vi "ReCalc_V0.16.vi"(3 "Berechnen":bool, 4 "Datenspeicher":T2={"Fahrzeugdaten"="", "date/time string"="", "Rolle [Inkr/U]"=0, "Rollenumfang [m]"=0.0, "Rollenträgheit [kgm²]"=0.0, "Zündung [Imp/U]"=0, "Getriebe [1:]"=0.0, "Reifenumfang [m] "=0.0, "element"=0.0, "Gl. Mittelwert"=0, "Differenzenquotient"=0, "Polynom"=0, "element"=0.0, "element"=0.0, "Lufttemperatur [°C]"=0.0, "Luftfeuchtigkeit [%]"=0.0, "Luftdruck [mbar]"=0.0, [], [], "Best Polynomial Fit"=[], [], "Übersetzung ermitteln aus"=0, "[s]"=0.0, "nmin [1/min]"=0.0, "nmax [1/min]"=0.0, "n vom Gas [1/min]"=0.0, [], [], "Boolesch"=FALSE, "Serielle Schnittstelle"="COM4"}) -> ()   [LabVIEW 2014]
uses:
  <vilib>/Utility/miscctls.llb/LVPointTypeDef.ctl
  <vilib>/Utility/xml.llb/Read From XML File(string).vi
  <vilib>/Analysis/3filter.llb/IIR Filter (DBL).vi
  <vilib>/Analysis/NI_AALBase.lvlib
  <vilib>/Analysis/NI_AALPro.lvlib
panel:
  out "Fahrzeugdaten":string
  out "Überlagerung":bool
  in  "Überlagern":bool
  out "Übersetzung ermitteln aus":T1(ring)
  in  "Speichern":bool
  out "Reifenumfang [m]":dbl=1.222
  out "Getriebe [1:]":dbl=5.343
  out "Zündung [Imp/U]":u8=1
  out "Rollengeber [Inkr/U]":u16=200
  out "Luftdruck [mbar]":dbl=1013.0
  out "Luftfeuchtigkeit [%]":dbl=50.0
  out "Lufttemperatur [°C]":dbl=20.0
  in  "Stopp":bool
  in  "Rollenträgheit [kgm²]":dbl=0.402
  in  "Polynom":u8=15
  in  "Gl. Mittelwert":u8=35
  in  "Differenzenquotient":u8=12
  in  "n vom Gas [1/min]":dbl=5000.0
  out "Rollenumfang [m]":dbl=0.613 format="%.3f"
  out "Datum, Zeit":string
  out "Untersetzung aus:":dbl=2.68 format="%.2f"
  in  "Drucken":bool
  out "Pmax":string
  out "Ergebnis":string
  out "XY-Graph":cluster{dbl[], dbl[]}[](graph)
  in  "Öffnen":bool
  out "korr":dbl
  out "[s]":dbl=5.0
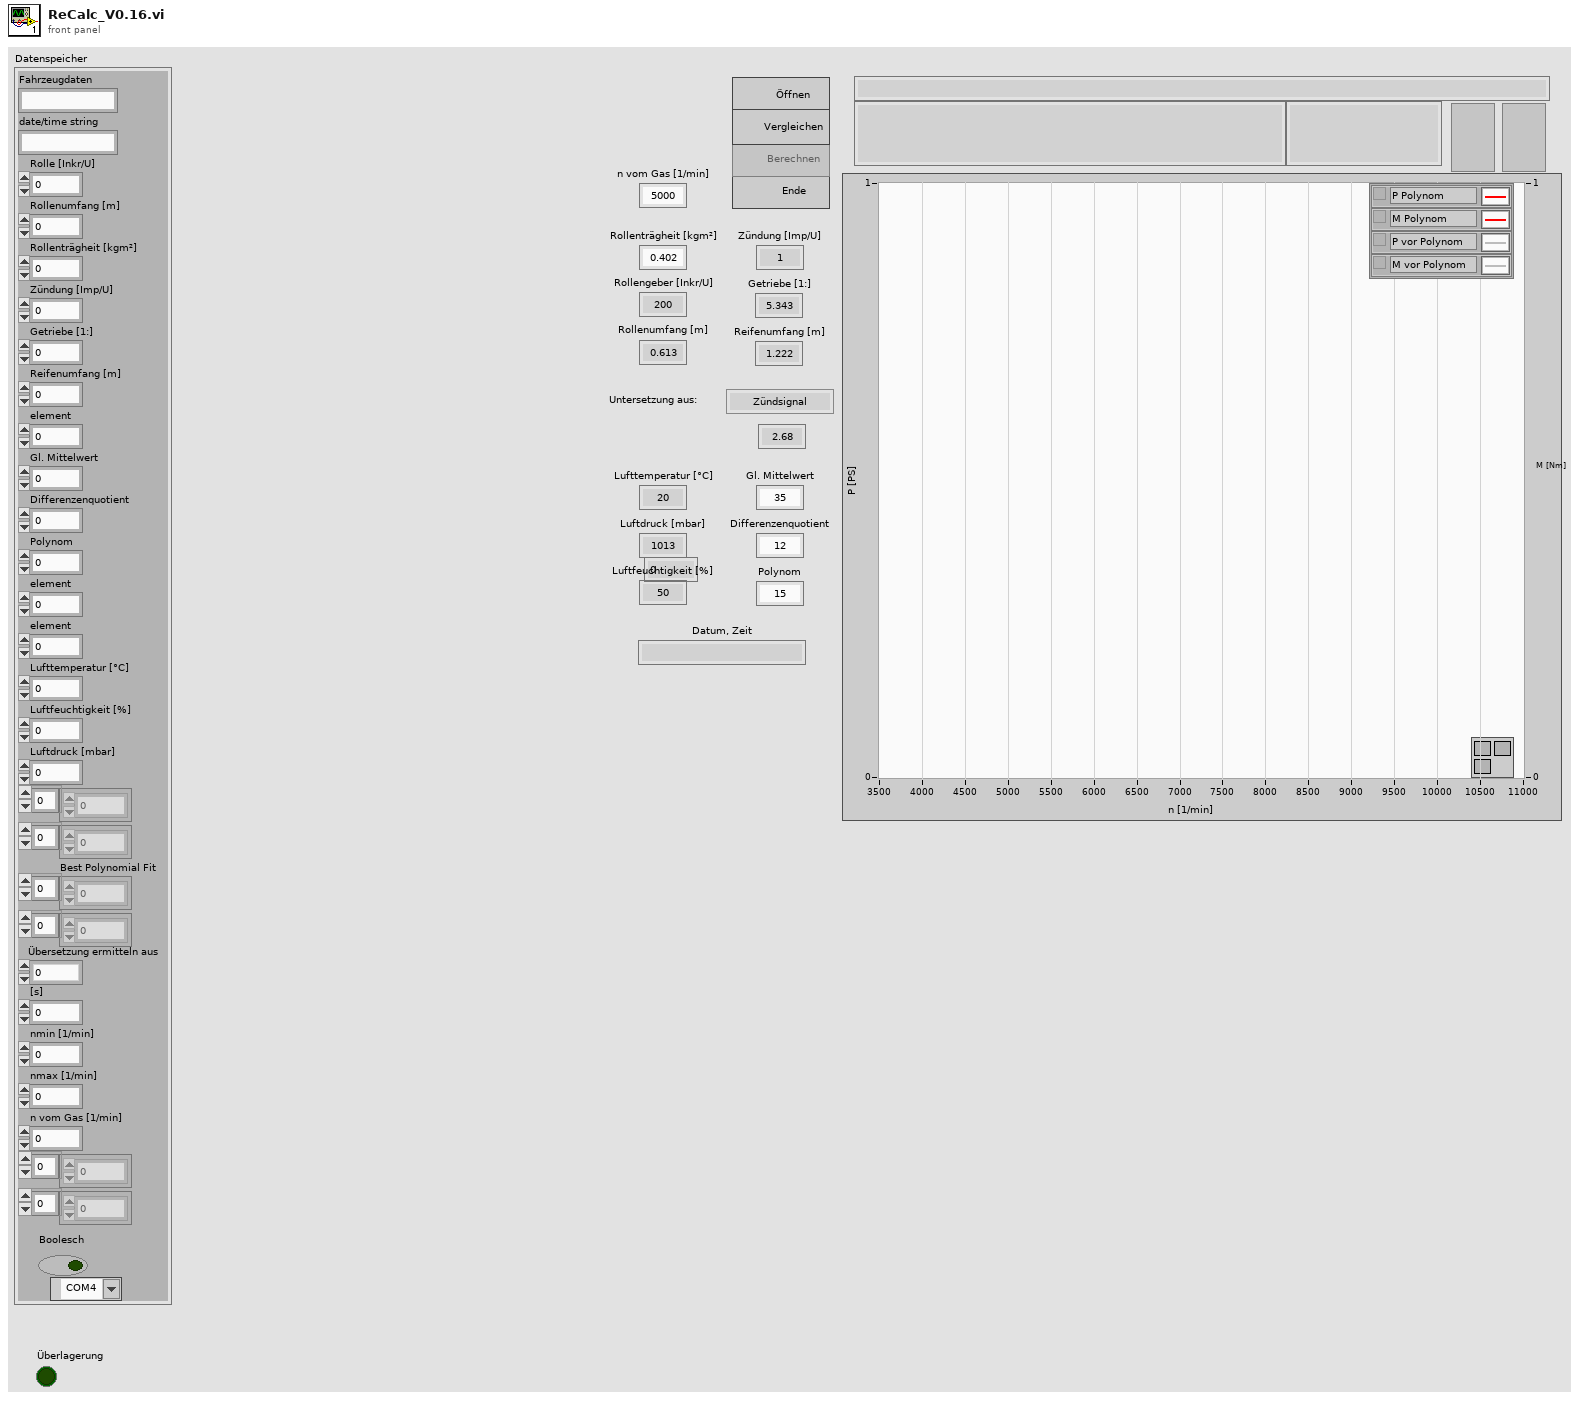
[diagram p1: front panel]
types:
  T1 = enum8{"Zündsignal", "Getriebe & Reifen", "nKuWe / nRolle :"}
  T2 = cluster{"Fahrzeugdaten":string, "date/time string":string, "Rolle [Inkr/U]":u16, "Rollenumfang [m]":dbl, "Rollenträgheit [kgm²]":dbl, "Zündung [Imp/U]":u8, "Getriebe [1:]":dbl, "Reifenumfang [m] ":dbl, "element":dbl, "Gl. Mittelwert":u8, "Differenzenquotient":u8, "Polynom":u8, "element":dbl, "element":dbl, "Lufttemperatur [°C]":dbl, "Luftfeuchtigkeit [%]":dbl, "Luftdruck [mbar]":dbl, dbl[], dbl[], "Best Polynomial Fit":dbl[], dbl[], "Übersetzung ermitteln aus":u8, "[s]":dbl, "nmin [1/min]":dbl, "nmax [1/min]":dbl, "n vom Gas [1/min]":dbl, dbl[], i32[], "Boolesch":bool, "Serielle Schnittstelle":refnum<visa-resource-name>}
  T3 = typedef "LVPointTypeDef.ctl" = cluster{"Horizontal":i16, "Vertical":i16}
  T4 = enum16{"Kleinste Quadrate", "Kleinestes absolutes Reiduum", "Biquadrat"}
  T5 = enum8{"Enabled", "Disabled", "Disabled and Grayed Out"}
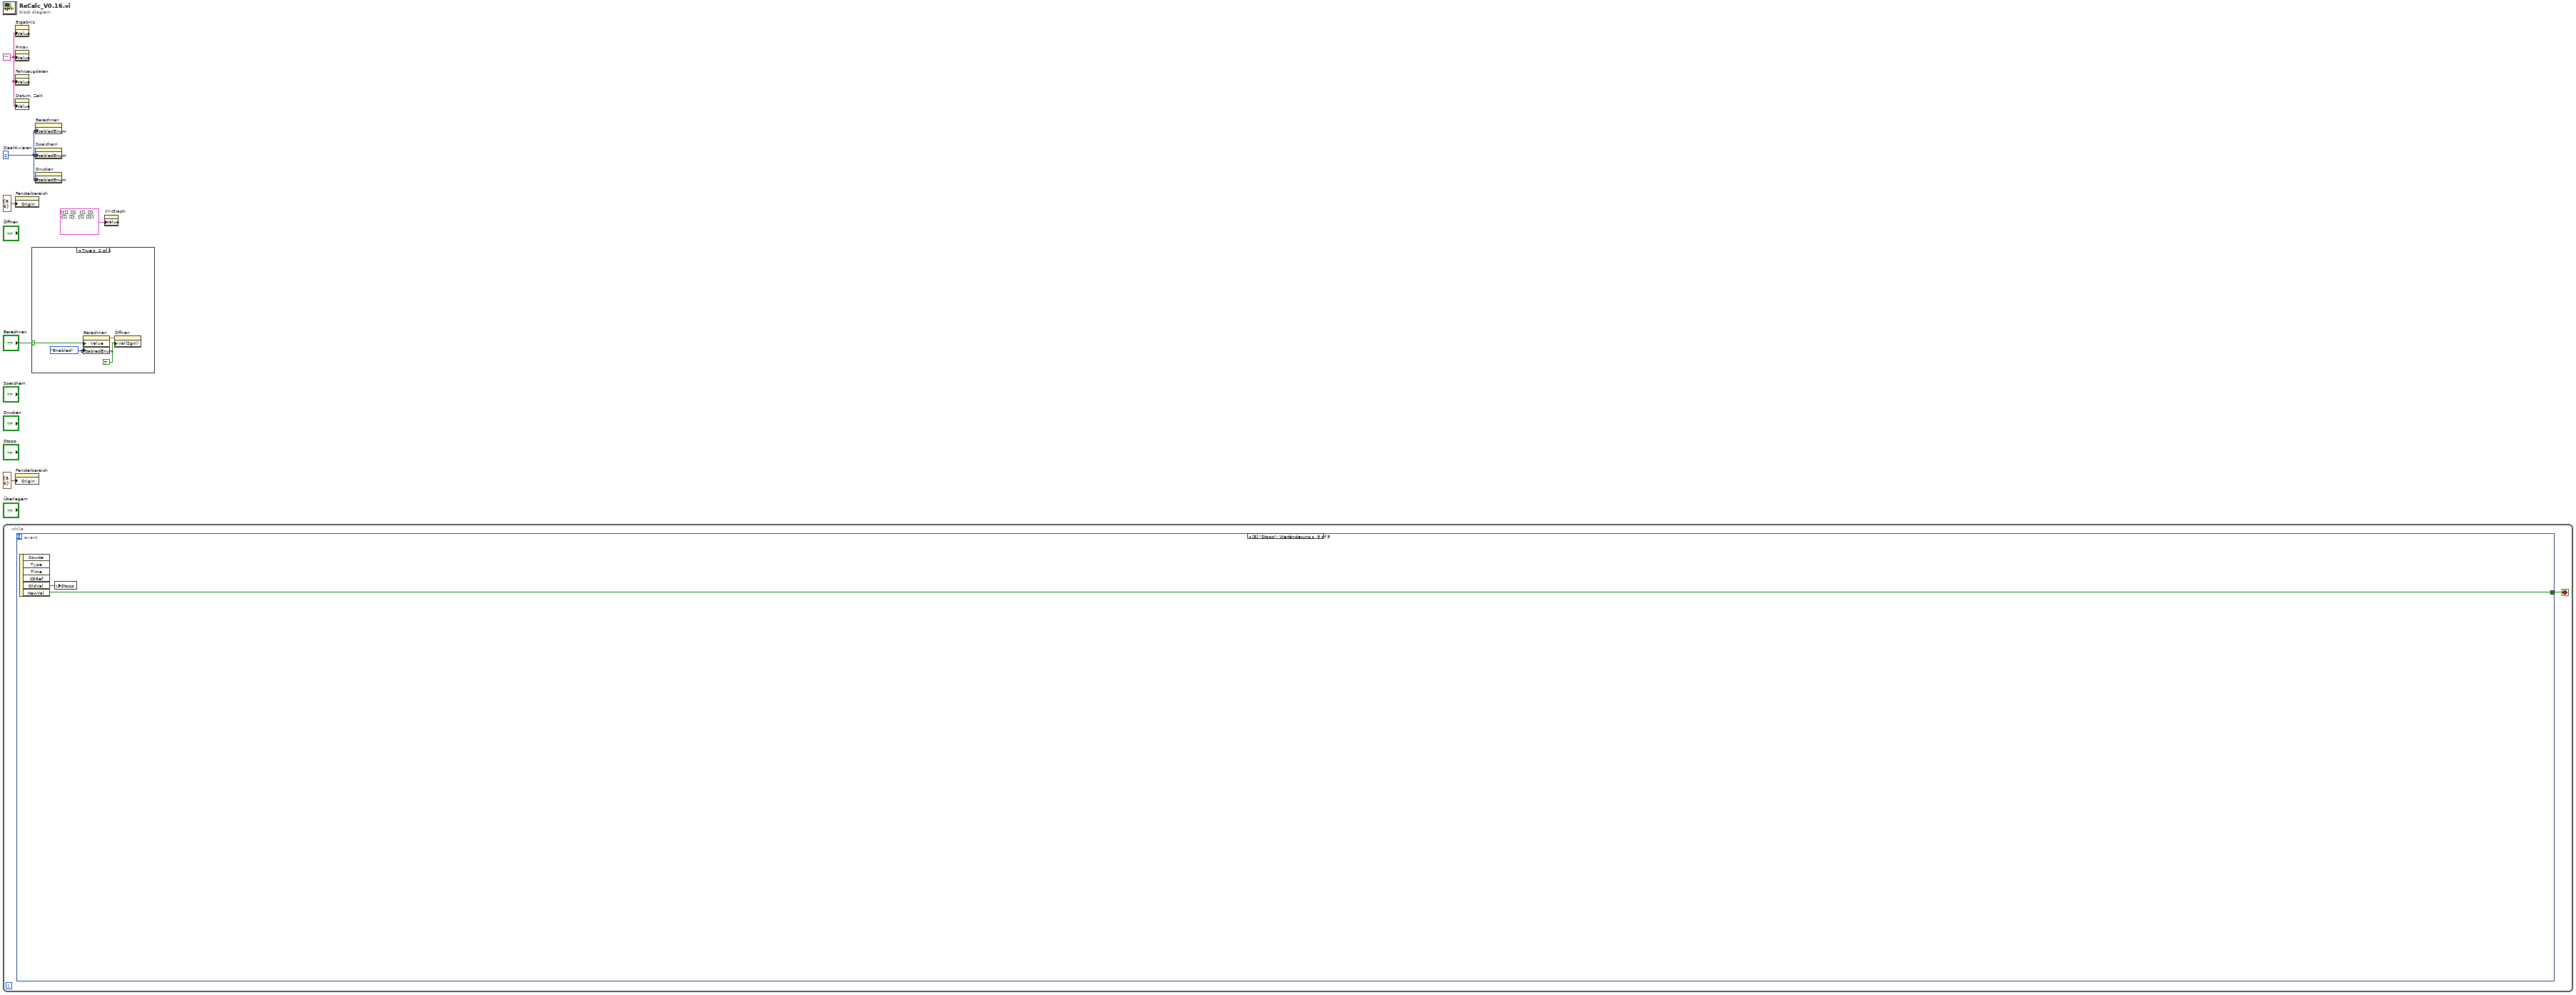
[diagram p0: block diagram]
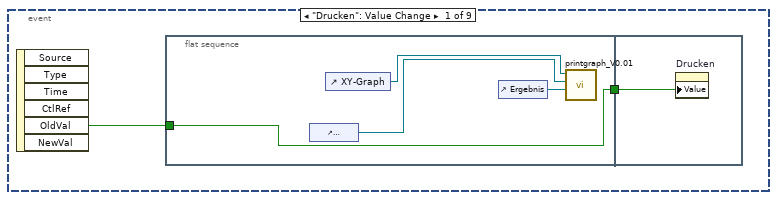
[diagram p3: hidden frame]
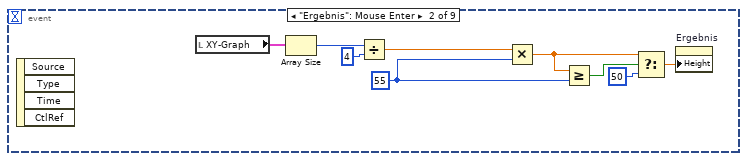
[diagram p4: hidden frame]
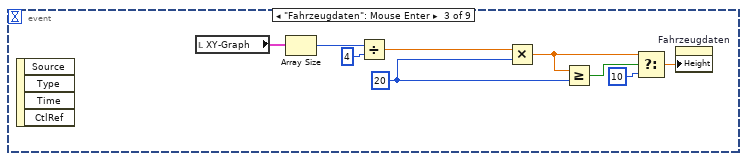
[diagram p5: hidden frame]
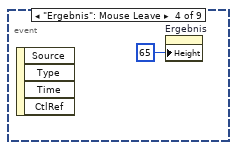
[diagram p6: hidden frame]
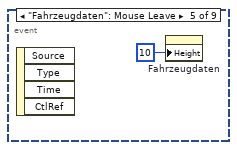
[diagram p7: hidden frame]
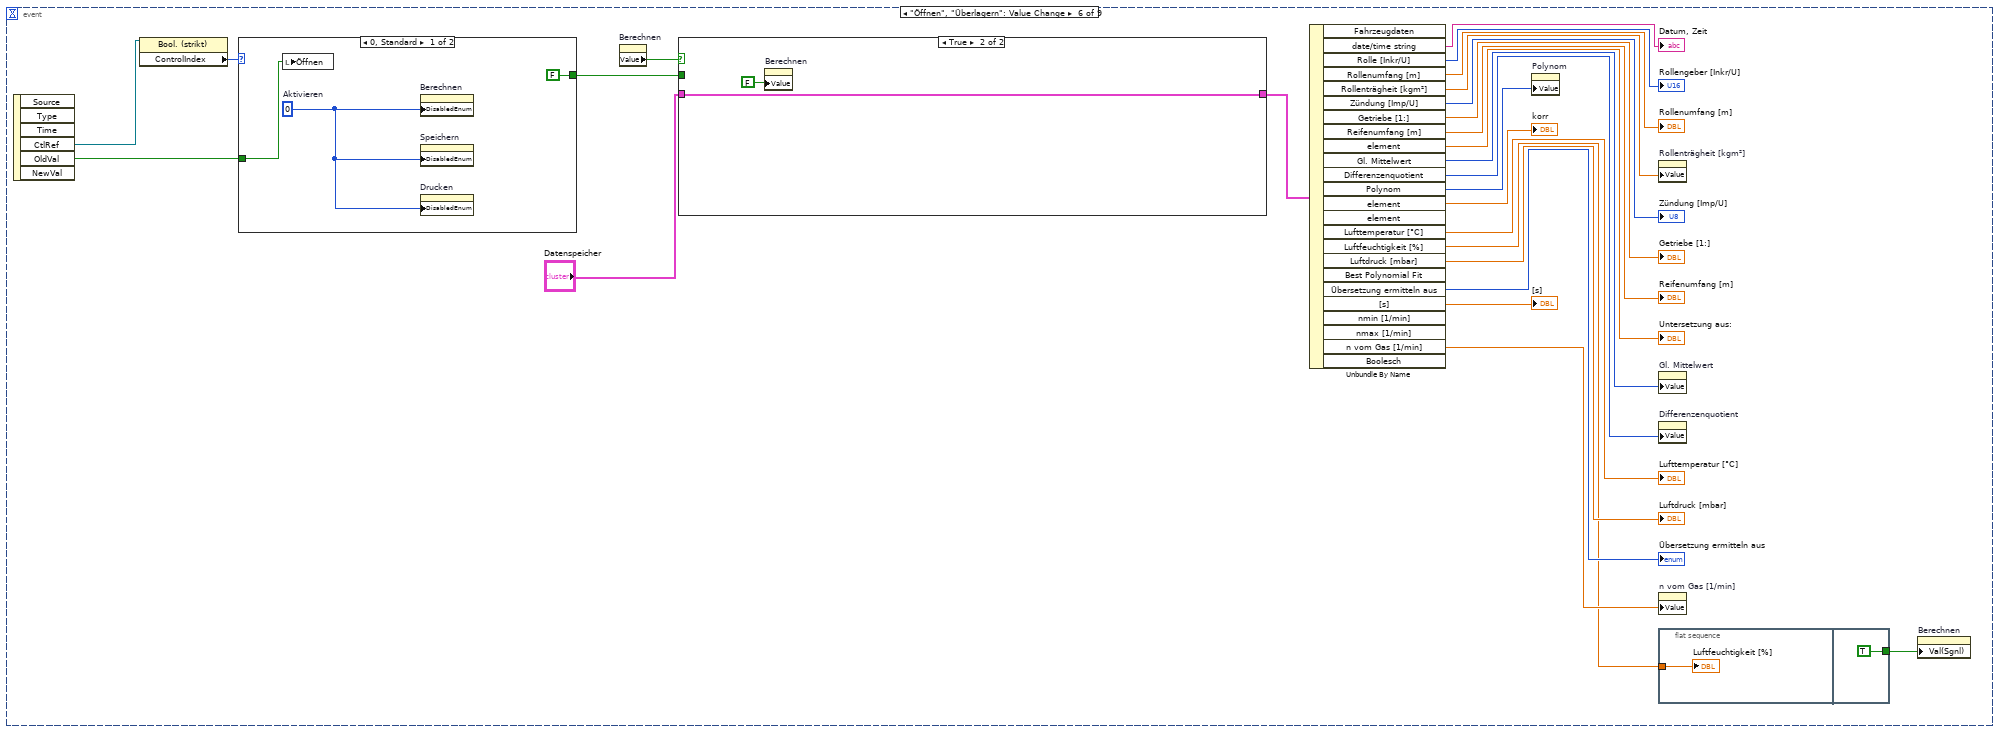
[diagram p8: hidden frame]
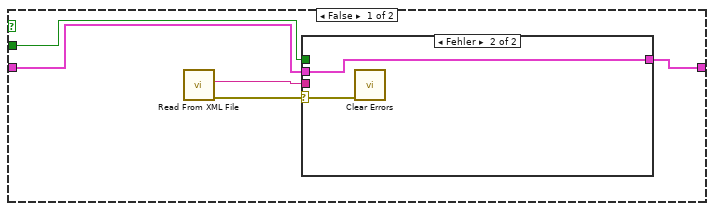
[diagram p9: hidden frame]
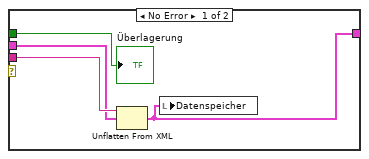
[diagram p10: hidden frame]
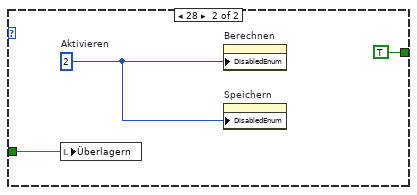
[diagram p11: hidden frame]
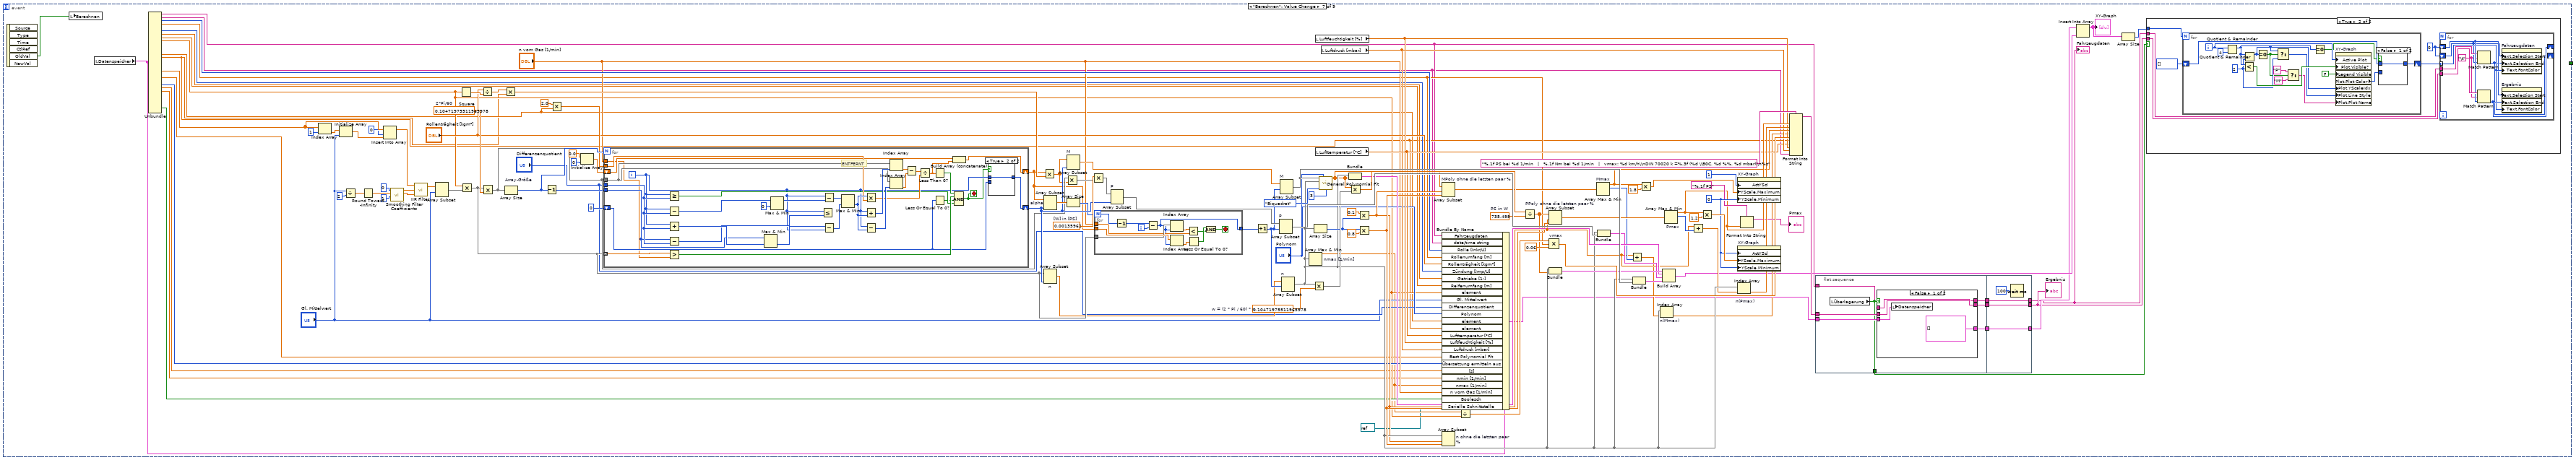
[diagram p12: hidden frame]
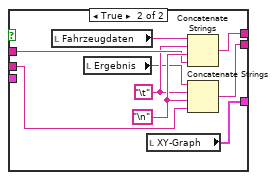
[diagram p13: hidden frame]
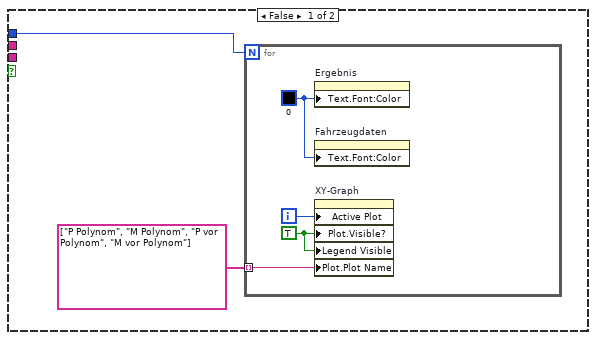
[diagram p14: hidden frame]
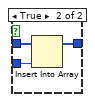
[diagram p15: hidden frame]
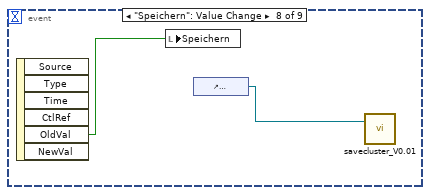
[diagram p17: hidden frame]
diagram:
  w4 = 2  # Deaktivieren
  w6 = ""
  n1 = while {
    stop <- w7 stop-if-true
    n2 = event shown="[8] \"Stopp\": Wertänderung" {
      selector: _ -> [_ _ _ _ _ _ _ _ _]
      dyn-events: _ -> [_ _ _ _ _ _ _ _ _]
      timeout: _ -> [_ _ _ _ _ _ _ _ _]
      tunnel: [_ _ _ _ _ _ _ _ w318] -> w7
      event "Drucken": Value Change {
        n3 = event-data() -> ("OldVal"=w9:bool)  [unwired: 1 in, 5 out]
        n4 = flat-sequence {
          tunnel: w9 -> [w13]
          tunnel: [w13] -> w8
          tunnel: w8 -> [w14]
          frame #0 {
            n5 = control-ref of="Fahrzeugdaten"() -> (w11:refnum<vi>)
            n6 = control-ref of="XY-Graph"() -> (w12:refnum<vi>)
            n7 = control-ref of="Ergebnis"() -> (w10:refnum<vi>)
            n8 = call "printgraph_V0.01.vi"("reference 2"=w10, "Fahrzeugdaten"=w11, "XYGraph (Eingang)"=w12) -> ()  [unwired: 9 in]
          }
          frame #1 {
            n9 = property on="Drucken" class="Bool. (strikt)"("Value"=w14) -> ()  [unwired: 2 in, 2 out]
          }
        }
      }
      event "Ergebnis": Mouse Enter {
        w17 = u32 55 ("Größe:Höhe")
        n10 = event-data() -> ()  [unwired: 1 in, 4 out]
        n11 = local read "XY-Graph"() -> (w23:cluster{dbl[], dbl[]}[])
        n12 = Array Size(array=w23) -> (size(s)=w22:i32)
        n13 = Divide(x=w22, y=4) -> (x/y=w20:dbl)
        n14 = Multiply(x=w20, y=w17) -> (x*y=w18:dbl)
        n15 = Greater Or Equal?(x=w18, y=w17) -> (x >= y?=w19:bool)
        n16 = Select(t=w18, s=w19, f=u32 50 ("Größe:Höhe")) -> (s? t:f=w16:dbl)
        n17 = property on="Ergebnis" class="Str"("Height"=w16) -> ()  [unwired: 2 in, 2 out]
      }
      event "Fahrzeugdaten": Mouse Enter {
        w26 = u32 20 ("Größe:Höhe")
        n18 = event-data() -> ()  [unwired: 1 in, 4 out]
        n19 = local read "XY-Graph"() -> (w32:cluster{dbl[], dbl[]}[])
        n20 = Array Size(array=w32) -> (size(s)=w31:i32)
        n21 = Divide(x=w31, y=4) -> (x/y=w29:dbl)
        n22 = Multiply(x=w29, y=w26) -> (x*y=w27:dbl)
        n23 = Greater Or Equal?(x=w27, y=w26) -> (x >= y?=w28:bool)
        n24 = Select(t=w27, s=w28, f=u32 10 ("Größe:Höhe")) -> (s? t:f=w25:dbl)
        n25 = property on="Fahrzeugdaten" class="Str"("Height"=w25) -> ()  [unwired: 2 in, 2 out]
      }
      event "Ergebnis": Mouse Leave {
        n26 = event-data() -> ()  [unwired: 1 in, 4 out]
        n27 = property on="Ergebnis" class="Str"("Height"=u32 65 ("Größe:Höhe")) -> ()  [unwired: 2 in, 2 out]
      }
      event "Fahrzeugdaten": Mouse Leave {
        n28 = event-data() -> ()  [unwired: 1 in, 4 out]
        n29 = property on="Fahrzeugdaten" class="Str"("Height"=u32 10 ("Größe:Höhe")) -> ()  [unwired: 2 in, 2 out]
      }
      event "Öffnen", "Überlagern": Value Change {
        n30 = event-data() -> ("CtlRef"=w59:refnum<vi>, "OldVal"=w57:bool)  [unwired: 1 in, 4 out]
        n31 = property class="Bool. (strikt)"(reference=w59) -> ("ControlIndex"=w58:i32)  [unwired: 1 in, 2 out]
        n32 = case shown="0, Standard" w58 {
          tunnel: w57 -> [w78 w81]
          tunnel: [FALSE ("Überlagerung") TRUE ("Überlagerung")] -> w56
          frame 0, Default {
            w76 = 0  # Aktivieren
            n33 = local write "Öffnen"(w78) -> ()
            n34 = property on="Berechnen" class="Bool. (strikt)"("DisabledEnum"=w76) -> ()  [unwired: 2 in, 2 out]
            n35 = property on="Speichern" class="Bool. (strikt)"("DisabledEnum"=w76) -> ()  [unwired: 2 in, 2 out]
            n36 = property on="Drucken" class="Bool. (strikt)"("DisabledEnum"=w76) -> ()  [unwired: 2 in, 2 out]
          }
          frame 28 {
            w79 = 2  # Aktivieren
            n37 = local write "Überlagern"(w81) -> ()
            n38 = property on="Berechnen" class="Bool. (strikt)"("DisabledEnum"=w79) -> ()  [unwired: 2 in, 2 out]
            n39 = property on="Speichern" class="Bool. (strikt)"("DisabledEnum"=w79) -> ()  [unwired: 2 in, 2 out]
          }
        }
        n40 = property on="Berechnen" class="Bool. (strikt)"() -> ("Value"=w35:bool)  [unwired: 2 in, 2 out]
        n41 = case shown="True" w35 {
          tunnel: "Datenspeicher" -> [w64 w72]
          tunnel: w56 -> [w62 _]
          tunnel: [w61 w72] -> w36
          frame False {
            n42 = call-poly <vilib>:"Read From XML File.vi"() -> ("error out"=w63:errorcluster, "XML Elements"=w65:string)  [unwired: 9 in, 1 out]
            n43 = case shown="Fehler" w63 {
              selector: w63 -> [_ w71]
              tunnel: w65 -> [w69 _]
              tunnel: w64 -> [w67 w70]
              tunnel: w62 -> [w68 _]
              tunnel: [w66 w70] -> w61
              frame No Error {
                n44 = Unflatten From XML(xml string=w69, type=w67) -> (value=w66:T2)  [unwired: 1 in, 1 out]
                n45 = local write "Datenspeicher"(w66) -> ()
                "Überlagerung" <- w68
              }
              frame Error {
                n46 = call <vilib>:"Clear Errors.vi"("error in (no error)"=w71) -> ()  [unwired: 5 in, 2 out]
              }
            }
          }
          frame True {
            n47 = property on="Berechnen" class="Bool. (strikt)"("Value"=FALSE) -> ()  [unwired: 2 in, 2 out]
          }
        }
        n48 = Unbundle By Name(w36) -> ("date/time string"=→"Datum, Zeit":string, "Rolle [Inkr/U]"=→"Rollengeber [Inkr/U]":u16, "Rollenumfang [m]"=→"Rollenumfang [m]":dbl, "Rollenträgheit [kgm²]"=w41:dbl, "Zündung [Imp/U]"=→"Zündung [Imp/U]":u8, "Getriebe [1:]"=→"Getriebe [1:]":dbl, "Reifenumfang [m]"=→"Reifenumfang [m]":dbl, "element"=→"Untersetzung aus:":dbl, "Gl. Mittelwert"=w46:u8, "Differenzenquotient"=w47:u8, "Polynom"=w48:u8, "element"=→"korr":dbl, "Lufttemperatur [°C]"=→"Lufttemperatur [°C]":dbl, "Luftfeuchtigkeit [%]"=w51:dbl, "Luftdruck [mbar]"=→"Luftdruck [mbar]":dbl, "Übersetzung ermitteln aus"=→"Übersetzung ermitteln aus":u8, "[s]"=→"[s]":dbl, "n vom Gas [1/min]"=w55:dbl)  [unwired: 6 out]
        n49 = property on="Polynom" class="DigWert (strikt)"("Value"=w48) -> ()  [unwired: 2 in, 2 out]
        n50 = property on="Rollenträgheit [kgm²]" class="DigWert (strikt)"("Value"=w41) -> ()  [unwired: 2 in, 2 out]
        n51 = property on="Gl. Mittelwert" class="DigWert (strikt)"("Value"=w46) -> ()  [unwired: 2 in, 2 out]
        n52 = property on="Differenzenquotient" class="DigWert (strikt)"("Value"=w47) -> ()  [unwired: 2 in, 2 out]
        n53 = property on="n vom Gas [1/min]" class="DigWert (strikt)"("Value"=w55) -> ()  [unwired: 2 in, 2 out]
        n54 = flat-sequence {
          tunnel: w51 -> [w74]
          tunnel: [TRUE] -> w37
          frame #0 {
            "Luftfeuchtigkeit [%]" <- w74
          }
          frame #1 {
          }
        }
        n55 = property on="Berechnen" class="Bool. (strikt)"("Val(Sgnl)"=w37) -> ()  [unwired: 2 in, 2 out]
      }
      event "Berechnen": Value Change {
        w165 = 0
        w173 = 735.498  # PS in W
        w178 = 0.10471975511965978  # w = (2 * Pi / 60) * n
        w189 = 0.00135962  # [W] in [PS]
        w198 = 0.10471975511965978  # 2*Pi/60
        n56 = event-data() -> ("OldVal"=w95:bool)  [unwired: 1 in, 5 out]
        n57 = local write "Berechnen"(w95) -> ()
        n58 = local read "Datenspeicher"() -> (w121:T2)
        n59 = Unbundle(w121) -> ("Fahrzeugdaten"=w87:string, "date/time string"=w86:string, "Rolle [Inkr/U]"=w117:u16, "Rollenumfang [m]"=w108:dbl, "Zündung [Imp/U]"=w107:u8, "Getriebe [1:]"=w106:dbl, "Reifenumfang [m]"=w105:dbl, "element"=w104:dbl, "element"=w103:dbl, "element"=w102:dbl, w204:dbl[], "Best Polynomial Fit"=w101:dbl[], "Übersetzung ermitteln aus"=w109:u8, "[s]"=w98:dbl, "nmin [1/min]"=w99:dbl, "Boolesch"=w112:bool)  [unwired: 14 out]
        n60 = Index Array(array=w204, index=1) -> (element=w127:dbl)
        n61 = Initialize Array(w127, "Gl. Mittelwert") -> (w128:dbl[])
        n62 = Divide(x="Gl. Mittelwert", y=2) -> (x/y=w201:dbl)
        n63 = Round Toward -Infinity(1:w201) -> (0:w200:dbl)
        n64 = Insert Into Array ("In Array einfügen")(array=w204, index=0, new element=w128) -> (w125:dbl[])
        n65 = call <vilib>:"Smoothing Filter Coefficients.vi"("shape"=1, "half-width"=w200, "type"=0) -> ("forward coefficients"=w129:dbl[], "reverse coefficients"=w130:dbl[])  [unwired: 6 in, 1 out]
        n66 = call-poly <vilib>:"IIR Filter.vi"("Forward Coefficients"=w129, "Reverse Coefficients"=w130, "X"=w125) -> ("Filtered X"=w124:dbl[])  [unwired: 1 in, 1 out]
        n67 = Array Subset(array=w124, index="Gl. Mittelwert") -> (w123:dbl[])  [unwired: 1 in]
        n68 = Square(x=w104) -> (x^2=w190:dbl)
        n69 = Multiply(x=w104, y=w123) -> (x*y=w132:dbl[])
        n70 = Divide(x="Rollenträgheit [kgm²]", y=w190) -> (x/y=w187:dbl)
        n71 = Multiply(x=w132, y=w198) -> (x*y=w155:dbl[])
        n72 = Multiply(x=w187, y=w102) -> (x*y=w186:dbl)
        n73 = Array Size "Array-Größe"(array=w155) -> (size(s)=w196:i32)
        n74 = Decrement(x=w196) -> (x-1=w197:i32)
        n75 = Multiply(x=2.0, y=w103) -> (x*y=w195:dbl)
        n76 = Initialize Array(0.0 ("y"), 0) -> (w191:dbl[])
        n77 = for {
          N: w196 -> [_]
          tunnel: "Differenzenquotient" -> [w291]
          tunnel: w155 -> [w298]
          tunnel: w197 -> [w290]
          tunnel: w195 -> [w299]
          shift-right: [w295] -> w154
          shift-left: w191 -> [w296]
          tunnel: w132 -> [w293] mode=indexing
          tunnel: "n vom Gas [1/min]" -> [w282]
          shift-right: [w281] -> w182
          shift-left: 0 -> [w284]
          i -> [w285]
          stop <- w283 stop-if-true
          # "ENTFERNT"
          n78 = Greater Or Equal?(x=w285, y=w291) -> (x >= y?=w288:bool)
          n79 = Subtract(x=w285, y=w291) -> (x-y=w312:i32)
          n80 = Add(x=w285, y=w291) -> (x+y=w306:i32)
          n81 = Subtract(x=w290, y=w291) -> (x-y=w292:i32)
          n82 = Greater?(x=w293, y=w282) -> (0:w294:bool)
          n83 = Max & Min(x=w290, y=w306) -> (min(x,y)=w307:i32)  [unwired: 1 out]
          n84 = Max & Min(x=w312, y=0) -> (max(x,y)=w310:i32)  [unwired: 1 out]
          n85 = Less Or Equal?(x=w285, y=w292) -> ()  [unwired: 1 out]
          n86 = Subtract(x=w285, y=w310) -> (x-y=w309:i32)
          n87 = Subtract(x=w307, y=w285) -> (x-y=w308:i32)
          n88 = Max & Min(x=w309, y=w308) -> (min(x,y)=w300:i32)  [unwired: 1 out]
          n89 = Multiply(x=w300, y=w299) -> (x*y=w297:dbl)
          n90 = Add(x=w285, y=w300) -> (x+y=w305:i32)
          n91 = Subtract(x=w285, y=w300) -> (x-y=w304:i32)
          n92 = Index Array(array=w298, index=w305) -> (element=w302:dbl)
          n93 = Index Array(array=w298, index=w304) -> (element=w303:dbl)
          n94 = Subtract(x=w302, y=w303) -> (x-y=w301:dbl)
          n95 = Divide(x=w301, y=w297) -> (x/y=w289:dbl)
          n96 = Less Than 0?(x=w289) -> (x < 0?=w287:bool)
          n97 = Less Or Equal To 0?(x=w284) -> (x <= 0?=w286:bool)
          n98 = Build Array (concatenate)(w296, w289) -> (w295:dbl[])
          n99 = Compound Arithmetic op=AND(w287, w294, w286, w288) -> (w283:bool)
          n100 = case shown="True" w283 {
            tunnel: w285 -> [_ w314]
            tunnel: [w313 w314] -> w281
            tunnel: w284 -> [w313 _]
            frame False {
            }
            frame True {
            }
          }
        }
        n101 = Multiply(x=w154, y=w186) -> (x*y=w152:dbl[])
        n102 = Array Subset "alpha"(array=w154, length=w182) -> (w184:dbl[])  [unwired: 1 in]
        n103 = Array Subset "n"(array=w132, length=w182) -> (w131:dbl[])  [unwired: 1 in]
        n104 = Multiply(x=w155, y=w152) -> (x*y=w188:dbl[])
        n105 = Array Subset "M"(array=w152, length=w182) -> (w153:dbl[])  [unwired: 1 in]
        n106 = Array Size(array=w184) -> (size(s)=w181:i32)
        n107 = Multiply(x=w189, y=w188) -> (x*y=w183:dbl[])
        n108 = for {
          N: w181 -> [w280]
          tunnel: w154 -> [w277]
          tunnel: w132 -> [w274]
          tunnel: "n vom Gas [1/min]" -> [w271]
          tunnel: [w269] -> w180
          i -> [w275]
          stop <- w270 stop-if-true
          n109 = Decrement(x=w280) -> (x-1=w279:i32)
          n110 = Subtract(x=w279, y=w275) -> (x-y=w269:i32)
          n111 = Index Array(array=w274, index=w269) -> (element=w273:dbl)
          n112 = Index Array(array=w277, index=w269) -> (element=w278:dbl)
          n113 = Less?(x=w273, y=w271) -> (x < y?=w272:bool)
          n114 = Less Or Equal To 0?(x=w278) -> (x <= 0?=w276:bool)
          n115 = And(x=w276, y=w272) -> (x .and. y?=w270:bool)
        }
        n116 = Array Subset "P"(array=w183, length=w182) -> (w172:dbl[])  [unwired: 1 in]
        n117 = Increment(x=w180) -> (x+1=w171:i32)
        n118 = Array Subset "P"(array=w172, index=w171) -> (w179:dbl[])  [unwired: 1 in]
        n119 = Array Subset "M"(array=w153, index=w171) -> (w177:dbl[])  [unwired: 1 in]
        n120 = Array Subset "n"(array=w131, index=w171) -> (w140:dbl[])  [unwired: 1 in]
        n121 = Array Max & Min "nmax [1/min]"(array=w140) -> (max value=w100:dbl)  [unwired: 3 out]
        n122 = Multiply(x=w140, y=w178) -> (x*y=w164:dbl[])
        n123 = Array Size(array=w140) -> (size(s)=w142:i32)
        n124 = local read "Luftfeuchtigkeit [%]"() -> (w119:dbl)
        n125 = local read "Lufttemperatur [°C]"() -> (w118:dbl)
        n126 = call <vilib>:"General Polynomial Fit.vi"("Y"=w177, "polynomial order"="Polynom", "X"=w140, "method"=T4."Biquadrat" ("Methode"), "algorithm"=3) -> ("Best Polynomial Fit"=w139:dbl[])  [unwired: 7 in, 3 out]
        n127 = local read "Luftdruck [mbar]"() -> (w120:dbl)
        n128 = Bundle(w140, "Best Polynomial Fit"=w139) -> (w150:cluster{dbl[], "Best Polynomial Fit":dbl[]})  [unwired: 1 in]
        n129 = Multiply(x=w139, y=w164) -> (x*y=w174:dbl[])
        n130 = Multiply(x=0.1, y=w142) -> (x*y=w135:dbl)
        n131 = Multiply(x=w142, y=0.8) -> (x*y=w143:dbl)
        n132 = Array Subset "MPoly ohne die letzten paar %"(array=w139, index=w135, length=w143) -> (w144:dbl[])
        n133 = Bundle By Name(cluster=w121, "Fahrzeugdaten"=w87, "date/time string"=w86, "Rolle [Inkr/U]"=w117, "Rollenumfang [m]"=w108, "Rollenträgheit [kgm²]"="Rollenträgheit [kgm²]", "Zündung [Imp/U]"=w107, "Getriebe [1:]"=w106, "Reifenumfang [m]"=w105, "element"=w104, "Gl. Mittelwert"="Gl. Mittelwert", "Differenzenquotient"="Differenzenquotient", "Polynom"="Polynom", "element"=w103, "element"=w102, "Lufttemperatur [°C]"=w118, "Luftfeuchtigkeit [%]"=w119, "Luftdruck [mbar]"=w120, "Best Polynomial Fit"=w101, "Übersetzung ermitteln aus"=w109, "[s]"=w98, "nmin [1/min]"=w99, "nmax [1/min]"=w100, "n vom Gas [1/min]"="n vom Gas [1/min]", "Boolesch"=w112, "Serielle Schnittstelle"=refnum<visa-resource-name> refnum) -> (w93:T2)
        n134 = Array Subset "n ohne die letzten paar %"(array=w140, index=w135, length=w143) -> ()  [unwired: 1 out]
        n135 = Divide(x=w100, y=w104) -> (x/y=w163:dbl)
        n136 = Divide(x=w174, y=w173) -> (x/y=w138:dbl[])
        n137 = Array Subset "PPoly ohne die letzten paar %"(array=w138, index=w135, length=w143) -> (w145:dbl[])
        n138 = Compound Arithmetic op=MULTIPLY "vmax"(w163, w108, 0.06) -> (w160:dbl)
        n139 = Bundle(w140, w138) -> (w151:cluster{dbl[], dbl[]})  [unwired: 1 in]
        n140 = Array Max & Min "Mmax"(array=w144) -> (max value=w157:dbl, max index (indices)=w136:i32)  [unwired: 2 out]
        n141 = Bundle(w140, w179) -> (w149:cluster{dbl[], dbl[]})  [unwired: 1 in]
        n142 = Add(x=w135, y=w136) -> (x+y=w134:dbl)
        n143 = Bundle(w140, w177) -> (w148:cluster{dbl[], dbl[]})  [unwired: 1 in]
        n144 = Multiply(x=w157, y=1.8) -> (x*y=w166:dbl)
        n145 = Index Array "n(Mmax)"(array=w140, index=w134) -> (element=w110:dbl)
        n146 = Build Array(w151, w150, w149, w148) -> (w91:cluster{dbl[], "Best Polynomial Fit":dbl[]}[])
        n147 = Array Max & Min "Pmax"(array=w145) -> (max value=w158:dbl, max index (indices)=w137:i32)  [unwired: 2 out]
        n148 = Add(x=w135, y=w137) -> (x+y=w133:dbl)
        n149 = Multiply(x=w158, y=1.2) -> (x*y=w167:dbl)
        n150 = property on="XY-Graph" class="XYGraph (strikt)"("ActYScl"=1, "YScale.Maximum"=w166, "YScale.Minimum"=w165) -> ()  [unwired: 2 in, 2 out]
        n151 = property on="XY-Graph" class="XYGraph (strikt)"("ActYScl"=w165, "YScale.Maximum"=w167, "YScale.Minimum"=w165) -> ()  [unwired: 2 in, 2 out]
        n152 = Index Array "n(Pmax)"(array=w140, index=w133) -> (element=w161:dbl)
        n153 = Format Into String(format string="%.1f PS" ("Format-String"), w158) -> (resulting string=→"Pmax":string)  [unwired: 2 in, 1 out]
        n154 = Format Into String(format string="%.1f PS bei %d 1/min   |   %.1f Nm bei %d 1/min   |   vmax: %d km/h\\nDIN 70020 k =%.3f (%d \\B0C, %d %%, %d mbar)\\n%s" ("Format-String"), w158, w161, w157, w110, w160, w102, w118, w119, w120, w86) -> (resulting string=w97:string)  [unwired: 2 in, 1 out]
        n155 = flat-sequence {
          tunnel: w97 -> [w211]
          tunnel: w93 -> [w210]
          tunnel: [w209] -> w92
          tunnel: w87 -> [w205]
          tunnel: [w208] -> w85
          tunnel: [w207] -> w84
          tunnel: [w206] -> w83
          tunnel: [w226] -> w88
          tunnel: [w227] -> w89
          tunnel: [w228] -> w90
          tunnel: w85 -> [w228]
          tunnel: w84 -> [w227]
          tunnel: w83 -> [w226]
          frame #0 {
            n156 = local read "Überlagerung"() -> (w209:bool)
            n157 = case shown="False" w209 {
              tunnel: [cluster{dbl[], dbl[]}[] [] ("XY-Graph") w224] -> w208
              tunnel: w211 -> [w214 w222]
              tunnel: [w214 w223] -> w207
              tunnel: w210 -> [w213 _]
              tunnel: w205 -> [w212 w220]
              tunnel: [w212 w219] -> w206
              frame False {
                n158 = local write "Datenspeicher"(w213) -> ()
              }
              frame True {
                w218 = "\t"
                w221 = "\n"
                n159 = local read "Fahrzeugdaten"() -> (w217:string)
                n160 = local read "Ergebnis"() -> (w216:string)
                n161 = local read "XY-Graph"() -> (w224:cluster{dbl[], dbl[]}[])
                n162 = Concatenate Strings(w217, w218, w221, w220) -> (w219:string)
                n163 = Concatenate Strings(w216, w218, w221, w222) -> (w223:string)
              }
            }
          }
          frame #1 {
            n164 = Wait (ms)(milliseconds to wait=u32 100 ("Zu wartende ms")) -> ()  [unwired: 1 out]
          }
        }
        n165 = Insert Into Array(array=w90, new element=w91) -> (w94:cluster{dbl[], dbl[]}[])  [unwired: 1 in]
        "XY-Graph" <- w94
        n166 = Array Size(array=w94) -> (size(s)=w96:i32)
        n167 = case shown="True" w92 {
          tunnel: w96 -> [w230 w240]
          tunnel: w89 -> [_ w237]
          tunnel: w88 -> [_ w236]
          frame False {
            n168 = for {
              N: w230 -> [_]
              tunnel: string[] ["P Polynom", "M Polynom", "P vor Polynom", "M vor Polynom"] -> [w232] mode=indexing
              i -> [w234]
              w231 = u32 0
              w233 = TRUE ("Plot.Sichtbar")
              n169 = property on="Ergebnis" class="Str"("Text.Font:Color"=w231) -> ()  [unwired: 2 in, 2 out]
              n170 = property on="Fahrzeugdaten" class="Str"("Text.Font:Color"=w231) -> ()  [unwired: 2 in, 2 out]
              n171 = property on="XY-Graph" class="XYGraph (strikt)"("Active Plot"=w234, "Plot.Visible?"=w233, "Legend Visible"=w233, "Plot.Plot Name"=w232) -> ()  [unwired: 2 in, 2 out]
            }
          }
          frame True {
            w235 = 0
            n172 = for {
              N: w240 -> [_]
              shift-right: [w259] -> w238
              shift-left: u32[] [] -> [w258]
              i -> [w263]
              w254 = 2 ("y")
              n173 = Quotient & Remainder(x=w263, y=4) -> (x-y*floor(x/y)=w256:i32)  [unwired: 1 out]
              n174 = Less?(x=w256, y=w254) -> (x < y?=w262:bool)
              n175 = Quotient & Remainder(x=w256, y=w254) -> (x-y*floor(x/y)=w255:i32)  [unwired: 1 out]
              n176 = Equal To 0?(x=w255) -> (x = 0?=w252:bool)
              n177 = Select(t=w255, s=w252, f=w254) -> (s? t:f=w253:i32)
              n178 = Select(t="P" ("Plot.Plotname"), s=w252, f="M" ("Plot.Plotname")) -> (s? t:f=w249:string)
              n179 = Equal To 0?(x=w256) -> (x = 0?=w257:bool)
              n180 = property on="XY-Graph" class="XYGraph (strikt)"("Active Plot"=w263, "Plot.Visible?"=w262, "Legend Visible"=FALSE ("Legende:Sichtbar"), "Plot.YScaleIdx"=w255, "Plot.Line Style"=w253, "Plot.Plot Name"=w249) -> ("Plot.Plot Color"=w260:u32)  [unwired: 2 in, 2 out]
              n181 = case shown="False" w257 {
                tunnel: w260 -> [_ w268]
                tunnel: [w265 w267] -> w259
                tunnel: w258 -> [w265 w266]
                frame False {
                }
                frame True {
                  n182 = Insert Into Array(array=w266, new element=w268) -> (w267:u32[])  [unwired: 1 in]
                }
              }
            }
            n183 = for {
              shift-right: [w248] -> _
              shift-left: w235 -> [w245]
              tunnel: w238 -> [w246] mode=indexing
              tunnel: w237 -> [w247]
              tunnel: w236 -> [w244]
              shift-right: [w243] -> _
              shift-left: w235 -> [w242]
              w241 = "\t"
              n184 = Match Pattern(string=w244, regular expression=w241, offset (0)=w242) -> (offset past match=w243:i32)  [unwired: 3 out]
              n185 = Match Pattern(string=w247, regular expression=w241, offset (0)=w245) -> (offset past match=w248:i32)  [unwired: 3 out]
              n186 = property on="Fahrzeugdaten" class="Str"("Text.Selection Start"=w242, "Text.Selection End"=w243, "Text.FontColor"=w246) -> ()  [unwired: 2 in, 2 out]
              n187 = property on="Ergebnis" class="Str"("Text.Selection Start"=w245, "Text.Selection End"=w248, "Text.FontColor"=w246) -> ()  [unwired: 2 in, 2 out]
            }
          }
        }
        "Ergebnis" <- w89
        "Fahrzeugdaten" <- w88
      }
      event "Speichern": Value Change {
        n188 = event-data() -> ("OldVal"=w316:bool)  [unwired: 1 in, 5 out]
        n189 = local write "Speichern"(w316) -> ()
        n190 = control-ref of="Datenspeicher"() -> (w315:refnum<vi>)
        n191 = call "savecluster_V0.01.vi"("Referenz"=w315) -> ()  [unwired: 2 in]
      }
      event "Stopp": Value Change {
        n192 = event-data() -> ("OldVal"=w317:bool, "NewVal"=w318:bool)  [unwired: 1 in, 4 out]
        n193 = local write "Stopp"(w317) -> ()
      }
    }
  }
  n194 = property on="Ergebnis" class="Str"("Value"=w6) -> ()  [unwired: 2 in, 2 out]
  n195 = property on="Pmax" class="Str"("Value"=w6) -> ()  [unwired: 2 in, 2 out]
  n196 = property on="Fahrzeugdaten" class="Str"("Value"=w6) -> ()  [unwired: 2 in, 2 out]
  n197 = property on="Datum, Zeit" class="Str"("Value"=w6) -> ()  [unwired: 2 in, 2 out]
  n198 = property on="Fensterbereich" class="Bereich"("Origin"=T3 {"Horizontal"=8, "Vertical"=6}) -> ()  [unwired: 2 in, 2 out]
  n199 = property on="Fensterbereich" class="Bereich"("Origin"=T3 {"Horizontal"=8, "Vertical"=6}) -> ()  [unwired: 2 in, 2 out]
  n200 = case shown="True" "Berechnen" {
    selector: "Berechnen" -> [_ w322]
    frame False {
    }
    frame True {
      n201 = property on="Berechnen" class="Bool. (strikt)"("Value"=w322, "DisabledEnum"=T5."Enabled" ("Deaktiviert")) -> (error out=w319:errorcluster)  [unwired: 2 in, 1 out]
      n202 = property on="Öffnen" class="Bool. (strikt)"(error in=w319, "Val(Sgnl)"=TRUE ("Wert (signalisierend)")) -> ()  [unwired: 1 in, 2 out]
    }
  }
  n203 = property on="Berechnen" class="Bool. (strikt)"("DisabledEnum"=w4) -> ()  [unwired: 2 in, 2 out]
  n204 = property on="Speichern" class="Bool. (strikt)"("DisabledEnum"=w4) -> ()  [unwired: 2 in, 2 out]
  n205 = property on="Drucken" class="Bool. (strikt)"("DisabledEnum"=w4) -> ()  [unwired: 2 in, 2 out]
  n206 = property on="XY-Graph" class="XYGraph (strikt)"("Value"=cluster{dbl[], dbl[]}[] [{[], []}, {[], []}, {[], []}, {[], []}] ("XY-Graph")) -> ()  [unwired: 2 in, 2 out]
